vi "del_trailing_zeros.vi"(10 "Array":dbl[](array[numeric])) -> (2 "Shortened array":dbl[](array[numeric]))   [LabVIEW 2014]
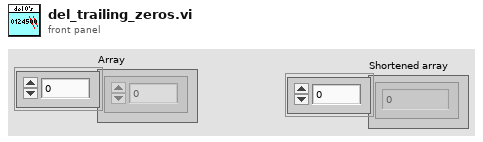
[diagram p1: front panel]
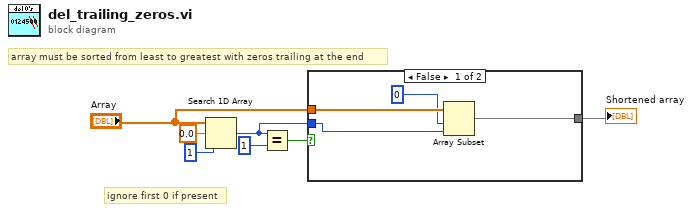
[diagram p0: block diagram]
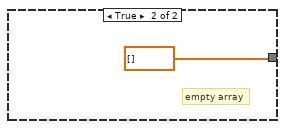
[diagram p2: hidden frame]
diagram:
  # "ignore first 0 if present"
  # "array must be sorted from least to greatest with zeros trailing at the end"
  n1 = Search 1D Array(1D array="Array", element=0.0, start index (0)=1) -> (index of element=w1:i32)
  n2 = Equal?(x=w1, y=1) -> (x = y?=w5:bool)
  n3 = case shown="False" w5 {
    tunnel: [w8 dbl[] []] -> w3
    tunnel: "Array" -> [w11 _]
    tunnel: w1 -> [w9 _]
    frame False {
      n4 = Array Subset(array=w11, index=0, length=w9) -> (w8:dbl[])
    }
    frame True {
      # "empty array"
    }
  }
  "Shortened array" <- w3
